vi "Configure Application Manager.vi"(8 "error in (no error)":errorcluster, 11 "TS UI Data in":T1) -> (0 "error out":errorcluster, 3 "TS UI Data out":T1)   [LabVIEW 2015]
uses:
  Type defs/TS UI Data.ctl
  Type defs/Nest cluster.ctl
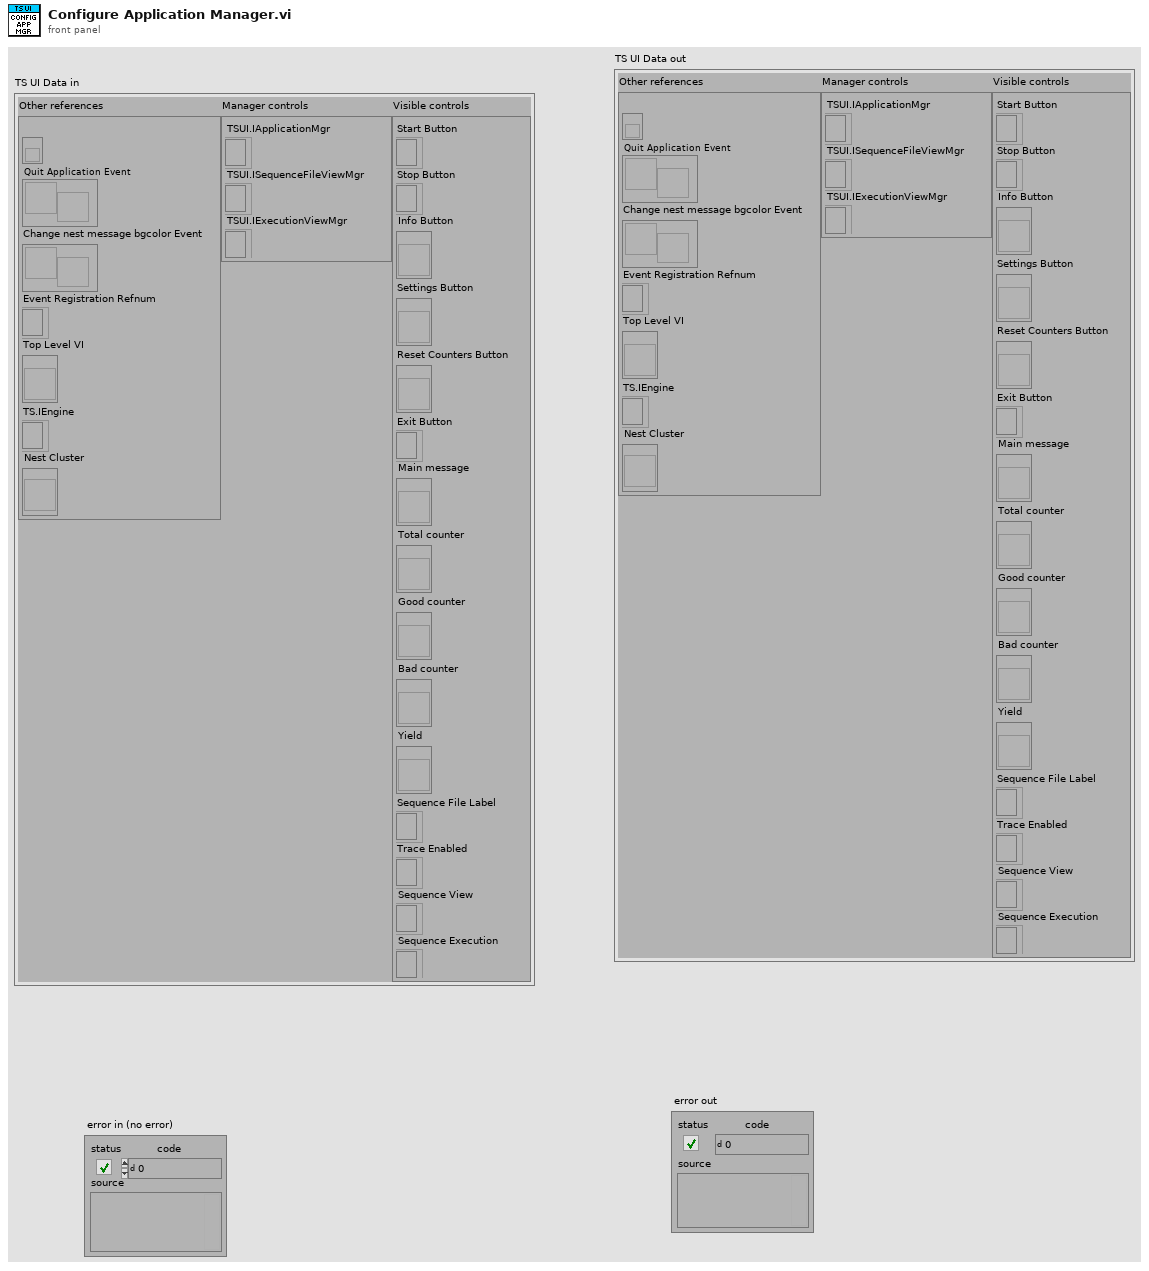
[diagram p1: front panel]
types:
  T1 = typedef "TS UI Data.ctl" = cluster{"Other references":cluster{"event callback refnum":refnum<k27>, "Quit Application Event":refnum<user-event>, "Change nest message bgcolor Event":refnum<user-event>, "event registration refnum":refnum<event-registration>, "Top Level VI":refnum<vi>, "TS.IEngine":refnum<k7>, "Nest Cluster":refnum<vi>}, "Manager controls":cluster{"TSUI.IApplicationMgr":refnum<k7>, "TSUI.ISequenceFileViewMgr":refnum<k7>, "TSUI.IExecutionViewMgr":refnum<k7>}, "Visible controls":cluster{"Start Button":refnum<k7>, "Stop Button":refnum<k7>, "Info Button":refnum<vi>, "Settings Button":refnum<vi>, "Reset Counters Button":refnum<vi>, "Exit Button":refnum<k7>, "Main message":refnum<vi>, "Total counter":refnum<vi>, "Good counter":refnum<vi>, "Bad counter":refnum<vi>, "Yield":refnum<vi>, "Sequence File Label":refnum<k7>, "Trace Enabled":refnum<k7>, "Sequence View":refnum<k7>, "Sequence Execution":refnum<k7>}}
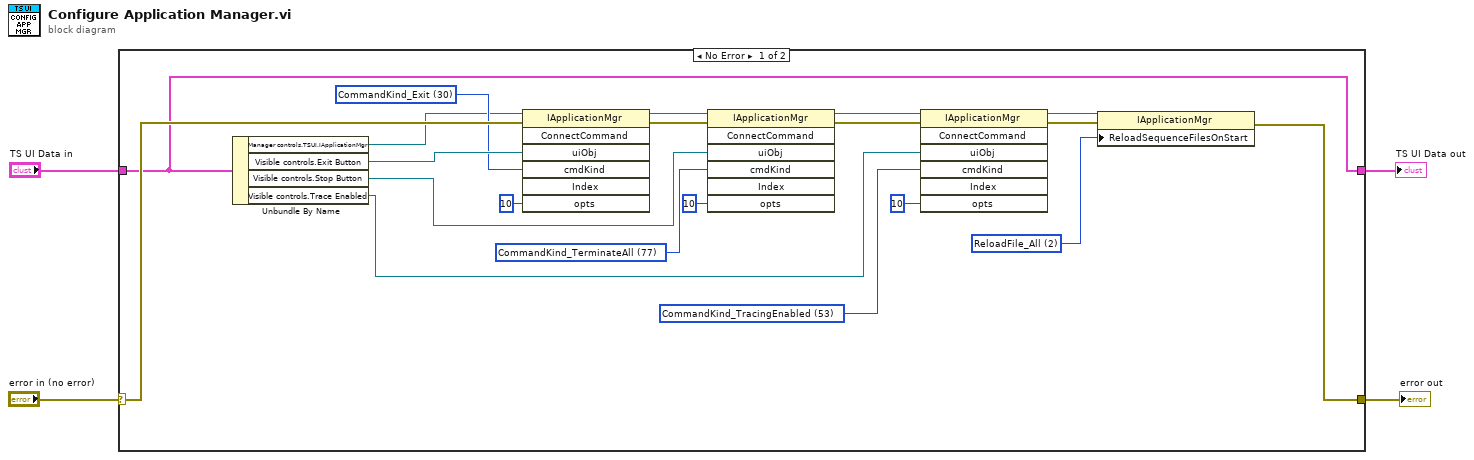
[diagram p0: block diagram]
diagram:
  n1 = case shown="No Error" "error in (no error)" {
    selector: "error in (no error)" -> [w24 w26]
    tunnel: "TS UI Data in" -> [w11 w25]
    tunnel: [w5 w26] -> w2
    tunnel: [w11 w25] -> w1
    frame No Error {
      w7 = 2 items=["ReloadFile_None", "ReloadFile_Selected", "ReloadFile_All"] ("ReloadSequenceFilesOnStart")
      w12 = 53 items=["CommandKind_NotACommand"=0, "CommandKind_Container"=1, "CommandKind_Separator"=2, "CommandKind_Custom"=3, "CommandKind_OpenSequenceFile"=20, "CommandKind_Close"=21, "CommandKind_CloseAll"=22, "CommandKind_CloseCompletedExecutions"=23, "CommandKind_OpenWorkspaceBrowser"=24, "CommandKind_Login"=25, "CommandKind_Logout"=26, "CommandKind_LoginLogout"=27, "CommandKind_UnloadAllModules"=28, "CommandKind_MRUFile"=29, "CommandKind_Exit"=30, "CommandKind_Restart"=40, "CommandKind_RunEntryPoint"=41, "CommandKind_RunEntryPointOnSelectedSteps"=42, "CommandKind_LoopEntryPointOnSelectedSteps"=43, "CommandKind_RunCurrentSequence"=44, "CommandKind_RunSpecificSequence"=45, "CommandKind_RunSelectedSteps"=46, "CommandKind_RunSelectedStepsUsingEntryPointsSubmenu"=47, "CommandKind_LoopOnSelectedSteps"=48, "CommandKind_LoopOnSelectedStepsUsingEntryPointsSubmenu"=49, "CommandKind_BreakOnFirstStep"=50, "CommandKind_BreakOnStepFailure"=51, "CommandKind_BreakOnSequenceFailure"=52, "CommandKind_TracingEnabled"=53, "CommandKind_ToggleBreakpoint"=60, "CommandKind_SetRunModeSubmenu"=61, "CommandKind_RunModeForcePass"=62, "CommandKind_RunModeForceFail"=63, "CommandKind_RunModeSkip"=64, "CommandKind_RunModeNormal"=65, "CommandKind_Resume"=66, "CommandKind_StepInto"=67, "CommandKind_StepOver"=68, "CommandKind_StepOut"=69, "CommandKind_SetNextStep"=70, "CommandKind_Break"=71, "CommandKind_BreakResume"=72, "CommandKind_Terminate"=73, "CommandKind_TerminateRestart"=74, "CommandKind_Abort"=75, "CommandKind_BreakAll"=76, "CommandKind_TerminateAll"=77, "CommandKind_AbortAll"=78, "CommandKind_ResumeAll"=79, "CommandKind_DisplayBreakpointsAndWatchExpressions"=80, "CommandKind_DisplayBreakpointSettings"=81, "CommandKind_BreakpointSubmenu"=85, "CommandKind_ConfigureAdapters"=90, "CommandKind_ConfigureStationOptions"=91, "CommandKind_ConfigureSearchDirectories"=92, "CommandKind_ConfigureExternalViewers"=93, "CommandKind_ToolItem"=100, "CommandKind_CustomizeTools"=101, "CommandKind_ExecutionEntryPointInsertionMarker"=110, "CommandKind_ExecutionEntryPointDefaultMenuInsertionMarker"=111, "CommandKind_ConfigurationEntryPointInsertionMarker"=112, "CommandKind_ConfigurationEntryPointDefaultMenuInsertionMarker"=113, "CommandKind_SequenceViewConfiguration"=116, "CommandKind_SequenceViewConfigurationsSubmenu"=118, "CommandKind_DefaultFileMenu_Set"=120, "CommandKind_DefaultExecuteMenu_Set"=121, "CommandKind_DefaultDebugMenu_Set"=123, "CommandKind_DefaultConfigureMenu_Set"=124, "CommandKind_DefaultToolsMenu_Set"=125, "CommandKind_DefaultSequenceViewContextMenu_Set"=126, "CommandKind_DefaultListBarContextMenu_Set"=127, "CommandKind_DefaultEditMenu_Set"=128, "CommandKind_DefaultSequenceListContextMenu_Set"=129, "CommandKind_SequenceViewConfigurations_Set"=139, "CommandKind_MRUFiles_Set"=140, "CommandKind_ExecutionEntryPoints_Set"=141, "CommandKind_RunSequences_Set"=142, "CommandKind_RunSelectedStepsUsingEntryPoints_Set"=143, "CommandKind_LoopOnSelectedStepsUsingEntryPoints_Set"=144, "CommandKind_ConfigurationEntryPoints_Set"=145, "CommandKind_Tools_Set"=146, "CommandKind_OpenSequenceFiles"=147, "CommandKind_LockUnlock"=148, "CommandKind_ConfigureSequenceViews"=149, "CommandKind_Edit_Undo"=200, "CommandKind_Edit_Redo"=201, "CommandKind_Edit_Rename"=202, "CommandKind_Edit_Cut"=203, "CommandKind_Edit_Copy"=204, "CommandKind_Edit_Paste"=205, "CommandKind_Edit_Delete"=206, "CommandKind_Edit_InsertStep"=207, "CommandKind_Edit_Save"=208, "CommandKind_Edit_SaveAs"=209, "CommandKind_Edit_SaveAll"=210, "CommandKind_Edit_NewSequenceFile"=211, "CommandKind_Edit_StepProperties"=212, "CommandKind_Edit_SequenceProperties"=213, "CommandKind_Edit_SequenceFileProperties"=214, "CommandKind_Edit_SpecifyModule"=215, "CommandKind_Edit_EditCode"=216, "CommandKind_Edit_EditStep"=217, "CommandKind_Edit_Preconditions"=218, "CommandKind_SelectAll"=219, "CommandKind_Edit_SelectDefaultAdapter"=220, "CommandKind_Edit_InsertSequence"=221, "CommandKind_Edit_SequenceFileCallbacks"=222, "CommandKind_Edit_EditPaths"=223, "CommandKind_Edit_EncapsulateSelectedSteps"=224, "CommandKind_Edit_InsertStepsSubmenu"=300, "CommandKind_Edit_EditStepsSubmenu"=301, "CommandKind_Edit_SelectDefaultAdaptersSubmenu"=302, "CommandKind_Edit_EncapsulateSelectedStepsSubmenu"=303, "CommandKind_Edit_InsertSteps_Set"=340, "CommandKind_Edit_EditSteps_Set"=341, "CommandKind_Edit_SelectDefaultAdapters_Set"=342, "CommandKind_Edit_EncapsulateSelectedSteps_Set"=343, "CommandKind_ShowInList"=400, "CommandKind_ShowInVariables"=401, "CommandKind_ShowTestStandHelp"=420, "CommandKind_ShowGuideToDocumentation"=421, "CommandKind_ShowHelpTopic"=422, "CommandKind_ShowTestStandWebResources"=423, "CommandKind_ShowTestStandDiscussionForum"=424, "CommandKind_ShowPatents"=425, "CommandKind_DefaultHelpMenu_Set"=440, "CommandKind_Edit_Attributes"=450, "CommandKind_Edit_AdvancedSequenceListSubmenu"=451, "CommandKind_ShowUpdateService"=452, "CommandKind_ShowExamples"=453, "CommandKind_ShowGettingStarted"=454] ("cmdKind")
      w17 = 77 items=["CommandKind_NotACommand"=0, "CommandKind_Container"=1, "CommandKind_Separator"=2, "CommandKind_Custom"=3, "CommandKind_OpenSequenceFile"=20, "CommandKind_Close"=21, "CommandKind_CloseAll"=22, "CommandKind_CloseCompletedExecutions"=23, "CommandKind_OpenWorkspaceBrowser"=24, "CommandKind_Login"=25, "CommandKind_Logout"=26, "CommandKind_LoginLogout"=27, "CommandKind_UnloadAllModules"=28, "CommandKind_MRUFile"=29, "CommandKind_Exit"=30, "CommandKind_Restart"=40, "CommandKind_RunEntryPoint"=41, "CommandKind_RunEntryPointOnSelectedSteps"=42, "CommandKind_LoopEntryPointOnSelectedSteps"=43, "CommandKind_RunCurrentSequence"=44, "CommandKind_RunSpecificSequence"=45, "CommandKind_RunSelectedSteps"=46, "CommandKind_RunSelectedStepsUsingEntryPointsSubmenu"=47, "CommandKind_LoopOnSelectedSteps"=48, "CommandKind_LoopOnSelectedStepsUsingEntryPointsSubmenu"=49, "CommandKind_BreakOnFirstStep"=50, "CommandKind_BreakOnStepFailure"=51, "CommandKind_BreakOnSequenceFailure"=52, "CommandKind_TracingEnabled"=53, "CommandKind_ToggleBreakpoint"=60, "CommandKind_SetRunModeSubmenu"=61, "CommandKind_RunModeForcePass"=62, "CommandKind_RunModeForceFail"=63, "CommandKind_RunModeSkip"=64, "CommandKind_RunModeNormal"=65, "CommandKind_Resume"=66, "CommandKind_StepInto"=67, "CommandKind_StepOver"=68, "CommandKind_StepOut"=69, "CommandKind_SetNextStep"=70, "CommandKind_Break"=71, "CommandKind_BreakResume"=72, "CommandKind_Terminate"=73, "CommandKind_TerminateRestart"=74, "CommandKind_Abort"=75, "CommandKind_BreakAll"=76, "CommandKind_TerminateAll"=77, "CommandKind_AbortAll"=78, "CommandKind_ResumeAll"=79, "CommandKind_DisplayBreakpointsAndWatchExpressions"=80, "CommandKind_DisplayBreakpointSettings"=81, "CommandKind_BreakpointSubmenu"=85, "CommandKind_ConfigureAdapters"=90, "CommandKind_ConfigureStationOptions"=91, "CommandKind_ConfigureSearchDirectories"=92, "CommandKind_ConfigureExternalViewers"=93, "CommandKind_ToolItem"=100, "CommandKind_CustomizeTools"=101, "CommandKind_ExecutionEntryPointInsertionMarker"=110, "CommandKind_ExecutionEntryPointDefaultMenuInsertionMarker"=111, "CommandKind_ConfigurationEntryPointInsertionMarker"=112, "CommandKind_ConfigurationEntryPointDefaultMenuInsertionMarker"=113, "CommandKind_SequenceViewConfiguration"=116, "CommandKind_SequenceViewConfigurationsSubmenu"=118, "CommandKind_DefaultFileMenu_Set"=120, "CommandKind_DefaultExecuteMenu_Set"=121, "CommandKind_DefaultDebugMenu_Set"=123, "CommandKind_DefaultConfigureMenu_Set"=124, "CommandKind_DefaultToolsMenu_Set"=125, "CommandKind_DefaultSequenceViewContextMenu_Set"=126, "CommandKind_DefaultListBarContextMenu_Set"=127, "CommandKind_DefaultEditMenu_Set"=128, "CommandKind_DefaultSequenceListContextMenu_Set"=129, "CommandKind_SequenceViewConfigurations_Set"=139, "CommandKind_MRUFiles_Set"=140, "CommandKind_ExecutionEntryPoints_Set"=141, "CommandKind_RunSequences_Set"=142, "CommandKind_RunSelectedStepsUsingEntryPoints_Set"=143, "CommandKind_LoopOnSelectedStepsUsingEntryPoints_Set"=144, "CommandKind_ConfigurationEntryPoints_Set"=145, "CommandKind_Tools_Set"=146, "CommandKind_OpenSequenceFiles"=147, "CommandKind_LockUnlock"=148, "CommandKind_ConfigureSequenceViews"=149, "CommandKind_Edit_Undo"=200, "CommandKind_Edit_Redo"=201, "CommandKind_Edit_Rename"=202, "CommandKind_Edit_Cut"=203, "CommandKind_Edit_Copy"=204, "CommandKind_Edit_Paste"=205, "CommandKind_Edit_Delete"=206, "CommandKind_Edit_InsertStep"=207, "CommandKind_Edit_Save"=208, "CommandKind_Edit_SaveAs"=209, "CommandKind_Edit_SaveAll"=210, "CommandKind_Edit_NewSequenceFile"=211, "CommandKind_Edit_StepProperties"=212, "CommandKind_Edit_SequenceProperties"=213, "CommandKind_Edit_SequenceFileProperties"=214, "CommandKind_Edit_SpecifyModule"=215, "CommandKind_Edit_EditCode"=216, "CommandKind_Edit_EditStep"=217, "CommandKind_Edit_Preconditions"=218, "CommandKind_SelectAll"=219, "CommandKind_Edit_SelectDefaultAdapter"=220, "CommandKind_Edit_InsertSequence"=221, "CommandKind_Edit_SequenceFileCallbacks"=222, "CommandKind_Edit_EditPaths"=223, "CommandKind_Edit_EncapsulateSelectedSteps"=224, "CommandKind_Edit_InsertStepsSubmenu"=300, "CommandKind_Edit_EditStepsSubmenu"=301, "CommandKind_Edit_SelectDefaultAdaptersSubmenu"=302, "CommandKind_Edit_EncapsulateSelectedStepsSubmenu"=303, "CommandKind_Edit_InsertSteps_Set"=340, "CommandKind_Edit_EditSteps_Set"=341, "CommandKind_Edit_SelectDefaultAdapters_Set"=342, "CommandKind_Edit_EncapsulateSelectedSteps_Set"=343, "CommandKind_ShowInList"=400, "CommandKind_ShowInVariables"=401, "CommandKind_ShowTestStandHelp"=420, "CommandKind_ShowGuideToDocumentation"=421, "CommandKind_ShowHelpTopic"=422, "CommandKind_ShowTestStandWebResources"=423, "CommandKind_ShowTestStandDiscussionForum"=424, "CommandKind_ShowPatents"=425, "CommandKind_DefaultHelpMenu_Set"=440, "CommandKind_Edit_Attributes"=450, "CommandKind_Edit_AdvancedSequenceListSubmenu"=451, "CommandKind_ShowUpdateService"=452, "CommandKind_ShowExamples"=453, "CommandKind_ShowGettingStarted"=454] ("cmdKind")
      w22 = 30 items=["CommandKind_NotACommand"=0, "CommandKind_Container"=1, "CommandKind_Separator"=2, "CommandKind_Custom"=3, "CommandKind_OpenSequenceFile"=20, "CommandKind_Close"=21, "CommandKind_CloseAll"=22, "CommandKind_CloseCompletedExecutions"=23, "CommandKind_OpenWorkspaceBrowser"=24, "CommandKind_Login"=25, "CommandKind_Logout"=26, "CommandKind_LoginLogout"=27, "CommandKind_UnloadAllModules"=28, "CommandKind_MRUFile"=29, "CommandKind_Exit"=30, "CommandKind_Restart"=40, "CommandKind_RunEntryPoint"=41, "CommandKind_RunEntryPointOnSelectedSteps"=42, "CommandKind_LoopEntryPointOnSelectedSteps"=43, "CommandKind_RunCurrentSequence"=44, "CommandKind_RunSpecificSequence"=45, "CommandKind_RunSelectedSteps"=46, "CommandKind_RunSelectedStepsUsingEntryPointsSubmenu"=47, "CommandKind_LoopOnSelectedSteps"=48, "CommandKind_LoopOnSelectedStepsUsingEntryPointsSubmenu"=49, "CommandKind_BreakOnFirstStep"=50, "CommandKind_BreakOnStepFailure"=51, "CommandKind_BreakOnSequenceFailure"=52, "CommandKind_TracingEnabled"=53, "CommandKind_ToggleBreakpoint"=60, "CommandKind_SetRunModeSubmenu"=61, "CommandKind_RunModeForcePass"=62, "CommandKind_RunModeForceFail"=63, "CommandKind_RunModeSkip"=64, "CommandKind_RunModeNormal"=65, "CommandKind_Resume"=66, "CommandKind_StepInto"=67, "CommandKind_StepOver"=68, "CommandKind_StepOut"=69, "CommandKind_SetNextStep"=70, "CommandKind_Break"=71, "CommandKind_BreakResume"=72, "CommandKind_Terminate"=73, "CommandKind_TerminateRestart"=74, "CommandKind_Abort"=75, "CommandKind_BreakAll"=76, "CommandKind_TerminateAll"=77, "CommandKind_AbortAll"=78, "CommandKind_ResumeAll"=79, "CommandKind_DisplayBreakpointsAndWatchExpressions"=80, "CommandKind_DisplayBreakpointSettings"=81, "CommandKind_BreakpointSubmenu"=85, "CommandKind_ConfigureAdapters"=90, "CommandKind_ConfigureStationOptions"=91, "CommandKind_ConfigureSearchDirectories"=92, "CommandKind_ConfigureExternalViewers"=93, "CommandKind_ToolItem"=100, "CommandKind_CustomizeTools"=101, "CommandKind_ExecutionEntryPointInsertionMarker"=110, "CommandKind_ExecutionEntryPointDefaultMenuInsertionMarker"=111, "CommandKind_ConfigurationEntryPointInsertionMarker"=112, "CommandKind_ConfigurationEntryPointDefaultMenuInsertionMarker"=113, "CommandKind_SequenceViewConfiguration"=116, "CommandKind_SequenceViewConfigurationsSubmenu"=118, "CommandKind_DefaultFileMenu_Set"=120, "CommandKind_DefaultExecuteMenu_Set"=121, "CommandKind_DefaultDebugMenu_Set"=123, "CommandKind_DefaultConfigureMenu_Set"=124, "CommandKind_DefaultToolsMenu_Set"=125, "CommandKind_DefaultSequenceViewContextMenu_Set"=126, "CommandKind_DefaultListBarContextMenu_Set"=127, "CommandKind_DefaultEditMenu_Set"=128, "CommandKind_DefaultSequenceListContextMenu_Set"=129, "CommandKind_SequenceViewConfigurations_Set"=139, "CommandKind_MRUFiles_Set"=140, "CommandKind_ExecutionEntryPoints_Set"=141, "CommandKind_RunSequences_Set"=142, "CommandKind_RunSelectedStepsUsingEntryPoints_Set"=143, "CommandKind_LoopOnSelectedStepsUsingEntryPoints_Set"=144, "CommandKind_ConfigurationEntryPoints_Set"=145, "CommandKind_Tools_Set"=146, "CommandKind_OpenSequenceFiles"=147, "CommandKind_LockUnlock"=148, "CommandKind_ConfigureSequenceViews"=149, "CommandKind_Edit_Undo"=200, "CommandKind_Edit_Redo"=201, "CommandKind_Edit_Rename"=202, "CommandKind_Edit_Cut"=203, "CommandKind_Edit_Copy"=204, "CommandKind_Edit_Paste"=205, "CommandKind_Edit_Delete"=206, "CommandKind_Edit_InsertStep"=207, "CommandKind_Edit_Save"=208, "CommandKind_Edit_SaveAs"=209, "CommandKind_Edit_SaveAll"=210, "CommandKind_Edit_NewSequenceFile"=211, "CommandKind_Edit_StepProperties"=212, "CommandKind_Edit_SequenceProperties"=213, "CommandKind_Edit_SequenceFileProperties"=214, "CommandKind_Edit_SpecifyModule"=215, "CommandKind_Edit_EditCode"=216, "CommandKind_Edit_EditStep"=217, "CommandKind_Edit_Preconditions"=218, "CommandKind_SelectAll"=219, "CommandKind_Edit_SelectDefaultAdapter"=220, "CommandKind_Edit_InsertSequence"=221, "CommandKind_Edit_SequenceFileCallbacks"=222, "CommandKind_Edit_EditPaths"=223, "CommandKind_Edit_EncapsulateSelectedSteps"=224, "CommandKind_Edit_InsertStepsSubmenu"=300, "CommandKind_Edit_EditStepsSubmenu"=301, "CommandKind_Edit_SelectDefaultAdaptersSubmenu"=302, "CommandKind_Edit_EncapsulateSelectedStepsSubmenu"=303, "CommandKind_Edit_InsertSteps_Set"=340, "CommandKind_Edit_EditSteps_Set"=341, "CommandKind_Edit_SelectDefaultAdapters_Set"=342, "CommandKind_Edit_EncapsulateSelectedSteps_Set"=343, "CommandKind_ShowInList"=400, "CommandKind_ShowInVariables"=401, "CommandKind_ShowTestStandHelp"=420, "CommandKind_ShowGuideToDocumentation"=421, "CommandKind_ShowHelpTopic"=422, "CommandKind_ShowTestStandWebResources"=423, "CommandKind_ShowTestStandDiscussionForum"=424, "CommandKind_ShowPatents"=425, "CommandKind_DefaultHelpMenu_Set"=440, "CommandKind_Edit_Attributes"=450, "CommandKind_Edit_AdvancedSequenceListSubmenu"=451, "CommandKind_ShowUpdateService"=452, "CommandKind_ShowExamples"=453, "CommandKind_ShowGettingStarted"=454] ("cmdKind")
      n2 = Unbundle By Name(w11) -> ("Manager controls.TSUI.IApplicationMgr"=w16:refnum<k7>, "Visible controls.Exit Button"=w23:refnum<k7>, "Visible controls.Stop Button"=w19:refnum<k7>, "Visible controls.Trace Enabled"=w13:refnum<k7>)
      n3 = invoke class="IApplicationMgr" method="ConnectCommand"(reference=w16, error in=w24, "uiObj"=w23, "cmdKind"=w22, "opts"=10) -> (reference out=w21:refnum<k7>, error out=w20:errorcluster)  [unwired: 2 in, 5 out]
      n4 = invoke class="IApplicationMgr" method="ConnectCommand"(reference=w21, error in=w20, "uiObj"=w19, "cmdKind"=w17, "opts"=10) -> (reference out=w15:refnum<k7>, error out=w14:errorcluster)  [unwired: 2 in, 5 out]
      n5 = invoke class="IApplicationMgr" method="ConnectCommand"(reference=w15, error in=w14, "uiObj"=w13, "cmdKind"=w12, "opts"=10) -> (reference out=w8:refnum<k7>, error out=w6:errorcluster)  [unwired: 2 in, 5 out]
      n6 = property class="IApplicationMgr"(reference=w8, error in=w6, "ReloadSequenceFilesOnStart"=w7) -> (error out=w5:errorcluster)  [unwired: 1 out]
    }
    frame Error {
    }
  }
  "error out" <- w2
  "TS UI Data out" <- w1
